vi "AVS_GetHandleFromSerial.vi"(0 "a_pSerial":i8) -> (4 "Output Value":i32)   [LabVIEW 2018]
uses:
  avaspecx64.dll
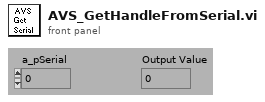
[diagram p1: front panel]
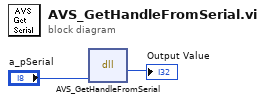
[diagram p0: block diagram]
diagram:
  n1 = dll-call lib="C:/AvaSpecX64-DLL_9.7/examples/LabView/LabViewSingleChan/avaspecx64.dll" fn="AVS_GetHandleFromSerial"("a_pSerial"="a_pSerial") -> ("return type"=→"Output Value":i32)  [unwired: 4 in, 2 out]
